vi "Scorer Post.vi"(8 "error in (no error)":errorcluster, 11 "Path":string="/scoring/next") -> (0 "error out":errorcluster, 2 "Status":i32, 3 "Content":string, 5 "Profile URL":string)   [LabVIEW 2024, in "Word Search Scorer.lvlib"]
uses:
  Word Search Scorer.lvlib
  Next Scoring Request.ctl
  <vilib>/httpClient/LabVIEWHTTPClient.lvlib
  <vilib>/httpClient/POSTBuffer.vi
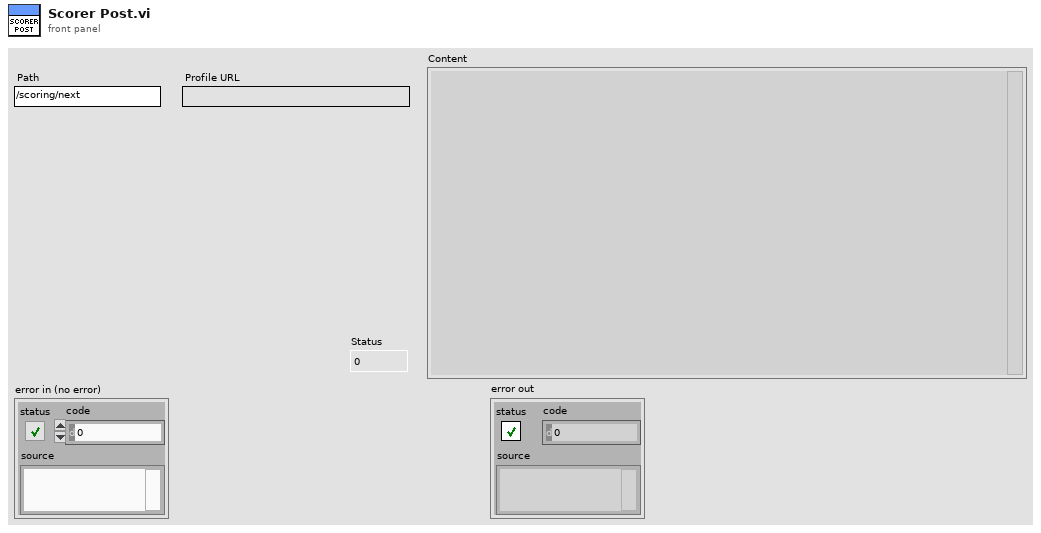
[diagram p1: front panel]
types:
  T1 = typedef "Word Search Scorer.lvlib/Next Scoring Request.ctl" = cluster{"scorer":string, "key":string, "challenges":i32[]}
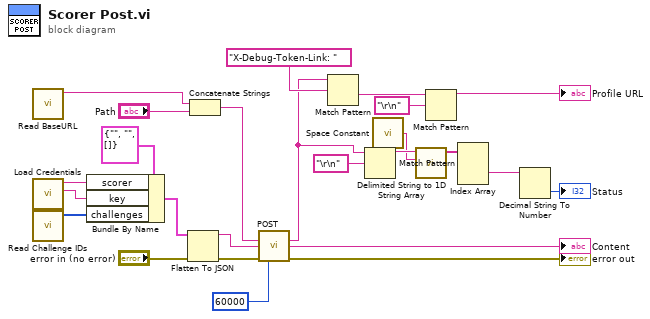
[diagram p0: block diagram]
diagram:
  n1 = call "Read BaseURL.vi"() -> ("BaseURL"=w12:string)  [unwired: 10 in, 1 out]
  n2 = call "Load Credentials.vi"() -> ("Key"=w17:string, "ID"=w24:string)  [unwired: 9 in, 1 out]
  n3 = call "Read Challenge IDs.vi"() -> ("IDs"=w23:i32[])  [unwired: 10 in, 1 out]
  n4 = Bundle By Name(cluster=T1 {"scorer"="", "key"="", "challenges"=[]} ("Next Scoring Request"), "scorer"=w24, "key"=w17, "challenges"=w23) -> (w22:T1)
  n5 = Flatten To JSON(anything=w22, error in (no error)="error in (no error)") -> (JSON string=w19:string, 11:w2:errorcluster)  [unwired: 1 in]
  n6 = Concatenate Strings(w12, "Path") -> (w20:string)
  n7 = call-poly <vilib>:"POST.vi"("url"=w20, "buffer"=w19, "error in (no error)"=w2, "timeout (10000)"=60000) -> ("headers"=w10:string, "body"=→"Content":string, "error out"=→"error out":errorcluster)  [unwired: 8 in, 1 out]
  n8 = Match Pattern(string=w10, regular expression="X-Debug-Token-Link: ") -> (after substring=w15:string)  [unwired: 1 in, 3 out]
  n9 = Match Pattern(string=w10, regular expression="\r\n") -> (before substring=w9:string)  [unwired: 1 in, 3 out]
  n10 = call <vilib>:"Space Constant.vi"() -> ("String"=w8:string)
  n11 = call <vilib>:"Delimited String to 1D String Array.vi"("delimiter"=w8, "delimited string"=w9) -> ("string array"=w7:string[])  [unwired: 9 in]
  n12 = Match Pattern(string=w15, regular expression="\r\n") -> (before substring=→"Profile URL":string)  [unwired: 1 in, 3 out]
  n13 = Index Array(array=w7) -> (element #2=w6:string)  [unwired: 3 in, 2 out]
  n14 = Decimal String To Number(string=w6) -> (number=→"Status":i32)  [unwired: 2 in, 1 out]
